vi "cSettingEventFunctionalGlobal.vi"(9 "cameraSettingsEventsRef":T1, 11 "Action":enum16{"Write", "Read"}(ring)) -> (1 "cameraSettingsEventsRef":T1)   [LabVIEW 2009, in "Tools.lvlib" / "Settings.lvlib"]
uses:
  Tools/Settings.lvlib
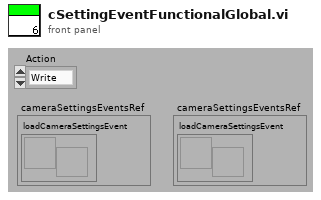
[diagram p1: front panel]
types:
  T1 = cluster{"loadCameraSettingsEvent":refnum<user-event>}
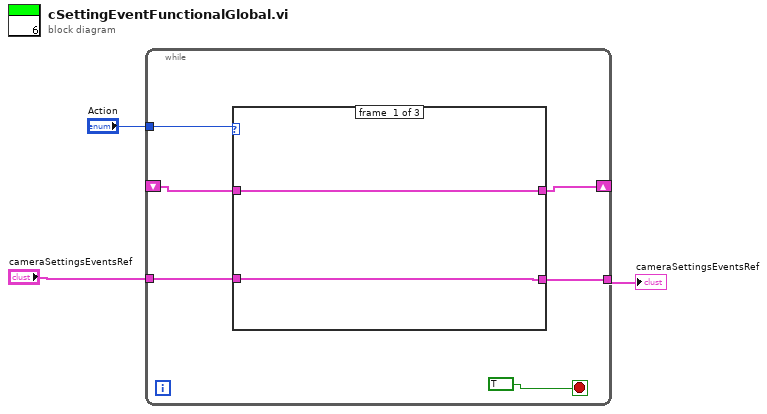
[diagram p0: block diagram]
diagram:
  n1 = while {
    tunnel: "Action" -> [w9]
    shift-right: [w4] -> _
    shift-left: _ -> [w6]
    tunnel: "cameraSettingsEventsRef" -> [w7]
    tunnel: [w5] -> w1
    stop <- TRUE stop-if-true
    n2 = case shown="\"Read\"" w9 {
      tunnel: [w11 w12 w13] -> w4
      tunnel: w7 -> [w10 w12 _]
      tunnel: w6 -> [w11 _ w13]
      tunnel: [w10 w12 w13] -> w5
      frame #0 {
      }
      frame #1 {
      }
      frame #2 {
      }
    }
  }
  "cameraSettingsEventsRef" <- w1
